vi "FFT x(t) to dB,Degrees_Ch3.VI"(11 "X(t)":dbl[](array[numeric]) format="%.2f") -> (0 "Nyquist Freq. Phase (degrees":dbl format="%.2f", 1 "Nyquist Freq. Mag (dB rms)":dbl format="%.2f", 2 "+Freq Phase of FFT (degrees)":dbl[](array[numeric]) format="%.2f", 3 "+Freq. Mag of FFT (dB rms)":dbl[](array[numeric]) format="%.2f", 4 "error":i32, 5 "+Freq Phase of FFT (radians)":dbl[](array[numeric]) format="%.2f", 6 "Nyquist Freq. Phase (radians)":dbl format="%.2f")   [LabVIEW 2015]
uses:
  <vilib>/Analysis/2dsp.llb/Real FFT.vi
  <vilib>/Analysis/NI_AALPro.lvlib
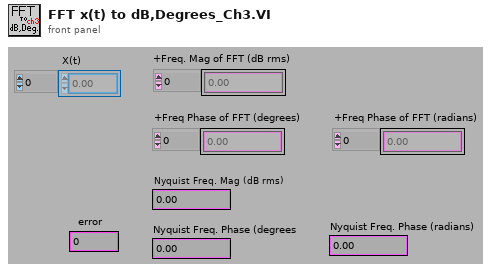
[diagram p1: front panel]
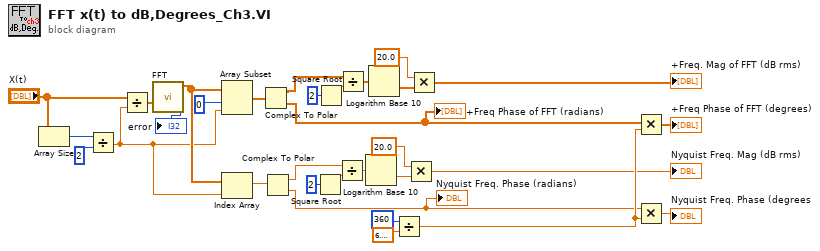
[diagram p0: block diagram]
diagram:
  n1 = Array Size(array="X(t)") -> (size(s)=w31:i32)
  n2 = Divide(x=w31, y=2) -> (x/y=w14:dbl)
  n3 = Divide(x="X(t)", y=w14) -> (x/y=w26:dbl[])
  n4 = call-poly <vilib>:"FFT.vi"("X"=w26) -> ("error"=→"error":i32, "FFT {X}"=w20:cdb[])  [unwired: 9 in]
  n5 = Array Subset(array=w20, index=0, length=w14) -> (w29:cdb[])
  n6 = Index Array(array=w20, index=w14) -> (element=w21:cdb)
  n7 = Complex To Polar(r * e^(i*theta)=w29) -> (r=w7:dbl[], theta=w2:dbl[])
  "+Freq Phase of FFT (radians)" <- w2
  n8 = Complex To Polar(r * e^(i*theta)=w21) -> (r=w4:dbl, theta=w1:dbl)
  "Nyquist Freq. Phase (radians)" <- w1
  n9 = Square Root(x=2) -> (sqrt(x)=w5:dbl)
  n10 = Square Root(x=2) -> (sqrt(x)=w8:dbl)
  n11 = Divide(x=w4, y=w5) -> (x/y=w3:dbl)
  n12 = Divide(x=w7, y=w8) -> (x/y=w10:dbl[])
  n13 = Logarithm Base 10(1:w3) -> (0:w18:dbl)
  n14 = Logarithm Base 10(1:w10) -> (0:w23:dbl[])
  n15 = Divide(x=360, y=6.283185307179586) -> (x/y=w13:dbl)
  n16 = Multiply(x=20.0, y=w18) -> (x*y=→"Nyquist Freq. Mag (dB rms)":dbl)
  n17 = Multiply(x=20.0, y=w23) -> (x*y=→"+Freq. Mag of FFT (dB rms)":dbl[])
  n18 = Multiply(x=w2, y=w13) -> (x*y=→"+Freq Phase of FFT (degrees)":dbl[])
  n19 = Multiply(x=w1, y=w13) -> (x*y=→"Nyquist Freq. Phase (degrees":dbl)
